vi "LVClass_ComputePhaseSet ctor from copy.vi"(0 "ComputePhaseSet in":refnum<class "ComputePhaseSet.lvclass">, 5 "ComputePhaseSet to copy in":refnum<class "ComputePhaseSet.lvclass">, 11 "error in (no error)":errorcluster) -> (4 "ComputePhaseSet out":refnum<class "ComputePhaseSet.lvclass">, 15 "error out":errorcluster)   [LabVIEW 2020, in "ComputePhaseSet.lvclass"]
doc: "ComputePhaseSet constructor from TypePhase value.\n\n--------------------------------------------------------------------------------\n\n<B>ComputePhaseSetIn </B> : Constant Pointer to ComputePhaseSet object.\n<B>ComputePhaseSetOut </B> : Constant Pointer to ComputePhaseSet object.\n<B>TypePhase </B> : TypePhase Polynomial bases enumeration.\n<B>ErrorIn </B> : Error\n<B>ErrorOut </B> : Error\n\n--------------------------------------------------------------------------------"
uses:
  ComputePhaseSet.lvclass
  WavefrontReconstructionMode.ctl
  Handle creation.ctl
  ComputePhaseSet.lvclass/ComputePhaseSet.ctl
  LVClass_ComputePhaseSet Read ComputePhaseSet.vi
panel:
  out "Reconstruction Mode":T1=enum."Modal_Legendre"
  out "ComputePhaseSet to copy out":refnum<class "ComputePhaseSet.lvclass">
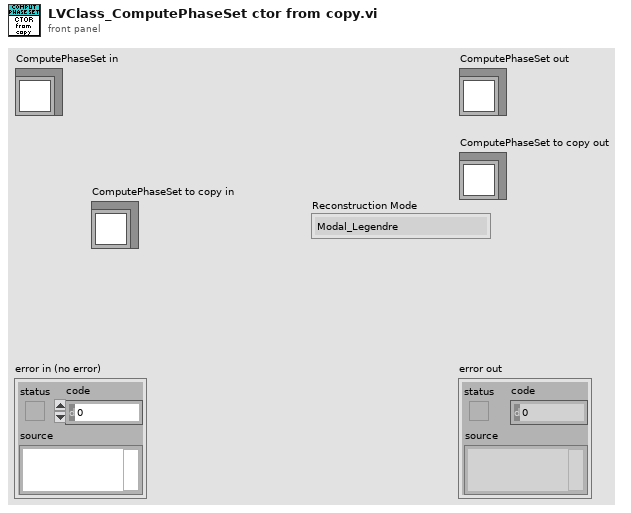
[diagram p1: front panel]
types:
  T1 = typedef "WavefrontReconstructionMode.ctl" = enum16{"None", "Modal_Legendre", "Modal_Zernike", "Zonal", "Modal_Zonal_Zernike", "Modal_Zonal_Legendre"}
  T2 = typedef "Handle creation.ctl" = enum16{"By ctor", "By write function"}
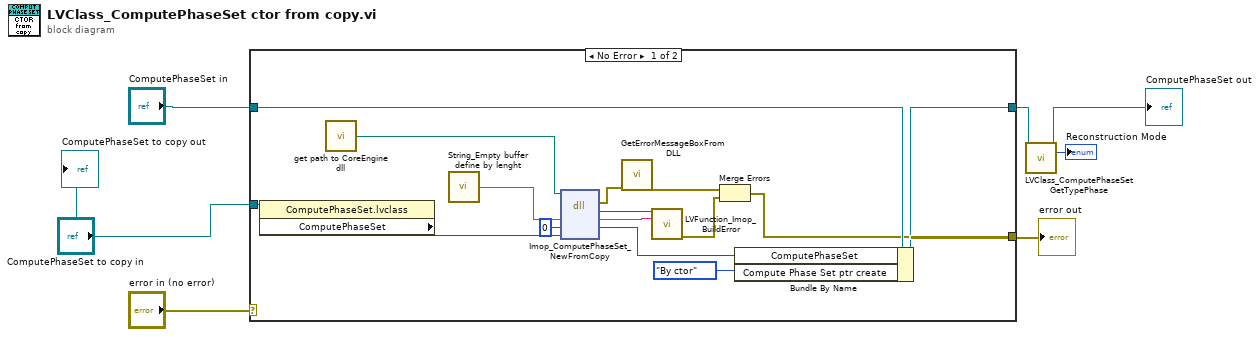
[diagram p0: block diagram]
diagram:
  n1 = case shown="No Error" "error in (no error)" {
    selector: "error in (no error)" -> [_ w24]
    tunnel: [w10 w24] -> w5
    tunnel: [w16 w23] -> w3
    tunnel: "ComputePhaseSet in" -> [w17 w23]
    tunnel: "ComputePhaseSet to copy in" -> [w9 _]
    frame No Error {
      n2 = property class="ComputePhaseSet.lvclass"(reference=w9) -> ("ComputePhaseSet"=w8:i32)  [unwired: 1 in, 2 out]
      n3 = call "get path to CoreEngine dll.vi"() -> ("path to c_interface_vc100.dll"=w14:path)  [unwired: 12 in, 3 out]
      n4 = call "String_Empty buffer define by lenght.vi"() -> ("Empty buffer"=w15:string)  [unwired: 1 in]
      n5 = dll-call lib="D:/soft/HASO_v3/SVN_trunk/ImOpCoreEngine4_LV2011/DLLs/c_interface_vc100.dll" fn="Imop_ComputePhaseSet_NewFromCopy"(path in=w14, "message"=w15, "objet"=0, "ComputePhaseSet_To_Copy"=w8) -> (error out=w13:errorcluster, "return type"=w20:i32, "message"=w19:string, "objet"=w18:i32)  [unwired: 3 in, 1 out]
      n6 = call "GetErrorMessageBoxFromDLL.vi"("error IN"=w13) -> ("error OUT"=w12:errorcluster)  [unwired: 10 in]
      n7 = call "LVFunction_Imop_BuildError.vi"("code"=w20, "String to Prepend to source (\"\")"=w19) -> ("error out"=w11:errorcluster)  [unwired: 13 in]
      n8 = Merge Errors(w12, w11) -> (w10:errorcluster)
      n9 = Bundle By Name(cluster=w17, "ComputePhaseSet"=w18, "Compute Phase Set ptr create"=Handle_creation."By ctor" ("Haso ptr create")) -> (w16:refnum<class "ComputePhaseSet.lvclass">)
    }
    frame Error {
    }
  }
  "error out" <- w5
  n10 = call "LVClass_ComputePhaseSet GetTypePhase.vi"("ComputePhaseSet in"=w3) -> ("ComputePhaseSet out"=→"ComputePhaseSet out":refnum<class "ComputePhaseSet.lvclass">, "Reconstruction Mode"=→"Reconstruction Mode":T1)  [unwired: 12 in, 1 out]
  "ComputePhaseSet to copy out" <- "ComputePhaseSet to copy in"
